vi "Scale singel variable.vi"(0 "Index":u16, 1 "Tool":bool, 7 "Val in":dbl, 11 "error in (no error)":errorcluster) -> (8 "Val out":dbl, 15 "error out":errorcluster)   [LabVIEW 2011]
uses:
  Common/Variable List Common Analog.ctl
  <vilib>/Utility/VariantDataType/GetNumericInfo.vi
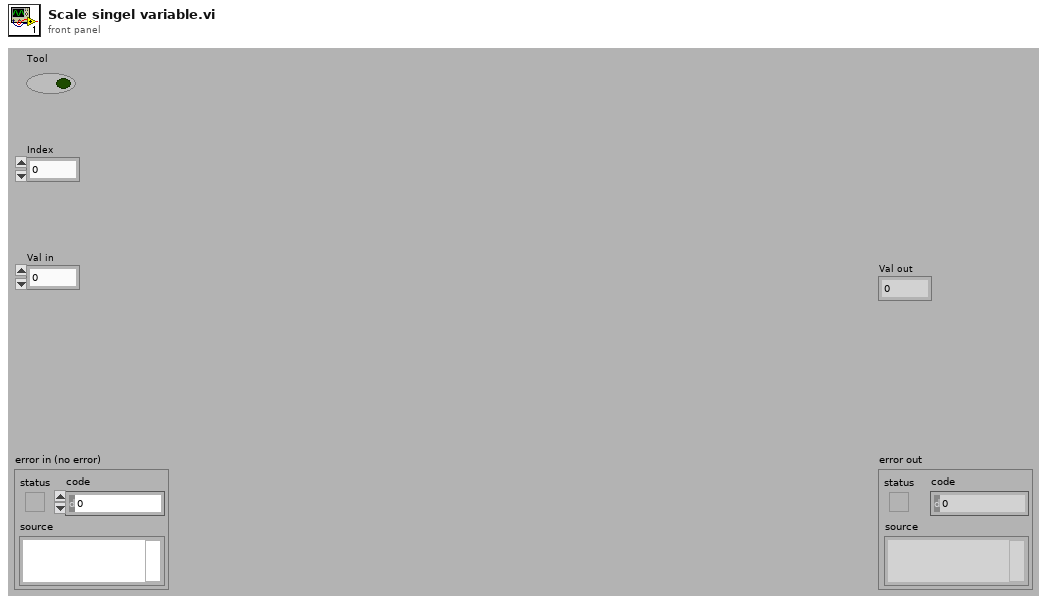
[diagram p1: front panel]
types:
  T1 = typedef "Variable List Common Analog.ctl" = enum16{"HVPSU Head Voltage", "HVPSU TS Voltage", "HVPSU Current", "PCP Cable Resistance", "Winch Depth", "Winch Line Speed", "Winch Wire Tension"}
  T2 = typedef "User Setting Analog Channel Bg.ctl" = cluster{"Scaling":T3, "Limits and responces":T4, "Allow Graph selection by user":bool, "Unit":u16}
  T3 = typedef "Scaling.ctl" = cluster{"Gain":dbl, "Offset":dbl}
  T4 = typedef "Alarm Setup Analog.ctl" = cluster{"Technical Error(NA)":T5, "LL":T5, "L":T5, "H":T5, "HH":T5, "Limits":T7}
  T5 = typedef "Alarm Responce.ctl" = cluster{"Action":T6, "Alarm":bool}
  T6 = typedef "Action List.ctl" = enum16{"No Action", "Stop Motor", "Turn Off HV"}
  T7 = typedef "Limits.ctl" = cluster{"LL":dbl, "L":dbl, "H":dbl, "HH":dbl}
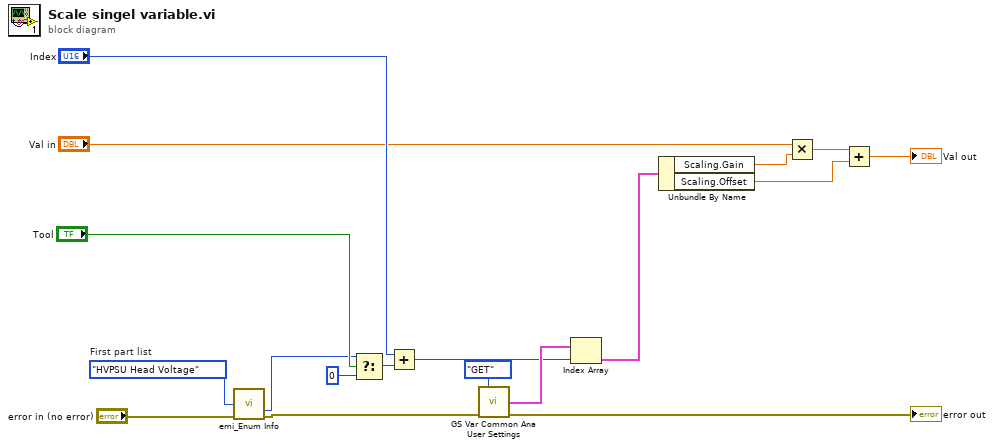
[diagram p0: block diagram]
diagram:
  w17 = Variable_List_Common_Analog."HVPSU Head Voltage"  # First part list
  n1 = call "emi_Enum Info.vi"("Enum"=w17, "error in (no error)"="error in (no error)") -> ("Numb Elements"=w15:i32, "error out"=w13:errorcluster)  [unwired: 10 in, 2 out]
  n2 = Select(t=w15, s="Tool", f=0) -> (s? t:f=w10:i32)
  n3 = Add(x="Index", y=w10) -> (x+y=w8:i32)
  n4 = call "GS Var Common Ana User Settings.vi"("Action(GET)"=enum16{"GET", "SET"}."GET", "error in (no error)"=w13) -> ("Common Analog var User set out"=w11:T2[], "error out"=→"error out":errorcluster)  [unwired: 11 in, 1 out]
  n5 = Index Array(array=w11, index=w8) -> (element=w6:T2)
  n6 = Unbundle By Name(w6) -> ("Scaling.Gain"=w5:dbl, "Scaling.Offset"=w2:dbl)
  n7 = Multiply(x="Val in", y=w5) -> (x*y=w3:dbl)
  n8 = Add(x=w3, y=w2) -> (x+y=→"Val out":dbl)
